vi "Global.vi"() -> ()   [LabVIEW 2020]
panel:
  out "Authorization":string
  out "产品进站":bool
  out "RecordDate":string
  out "接口调用频率":u32
  out "正在运行":bool
  out "待机超限时间":u32
  out "强制停止":bool
  out "MES状态":bool
  in  "MES参数":T1
  in  "运行状态位置":i32
  out "气密保持压力持续时间":string
  out "气密充气时间":string
  out "气密保持压力":string
  out "运行状态时间点":dbl[](array[numeric])
  out "PACK编码":string
  out "员工编号":string
  out "mes抬头":string[][](array[string])
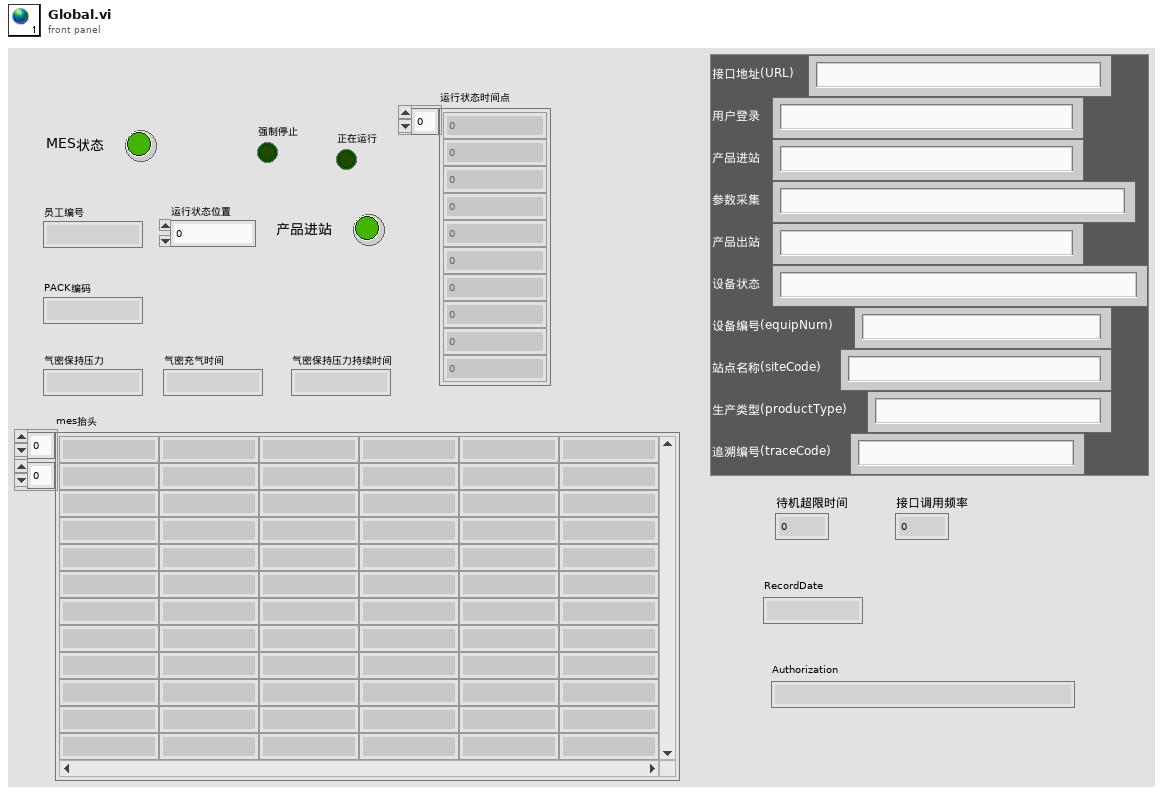
[diagram p1: front panel]
types:
  T1 = cluster{"接口地址(URL)":string, "用户登录":string, "产品进站":string, "参数采集":string, "产品出站":string, "设备状态":string, "设备编号(equipNum)":string, "站点名称(siteCode)":string, "生产类型(productType)":string, "追溯编号(traceCode)":string}
diagram:
